vi "OnDrop.vi"(0 "XRef":T8, 1 "State In":T1 {"BlockNodeState"."Draw Style" items=["FunctionBlock", "ExpressVI", "Variable", "Elemental I/O", "32x32 Icon", "FunctionBlockCompact"]; "BlockNodeState"."Terminal Data"."Terminal Flags" format="%.0b"}) -> (14 "Reply":T6, 16 "State Out":T1 {"BlockNodeState"."Draw Style" items=["FunctionBlock", "ExpressVI", "Variable", "Elemental I/O", "32x32 Icon", "FunctionBlockCompact"]; "BlockNodeState"."Terminal Data"."Terminal Flags" format="%.0b"})   [LabVIEW 2018, in "N9010A_SCPI Node.xnode"]
uses:
  N9010A_SCPI Node.xnode
  <vilib>/XNodeSupport/XNodeXNodeRef.ctl
  State.ctl
  <vilib>/BlockNodeSupport/BlockNodeState.ctl
  <vilib>/BlockNodeSupport/TerminalData.ctl
  <vilib>/picture/picture.llb/imagedata.ctl
  Utility/command_spec.ctl
  <vilib>/XNodeSupport/XNodeStringArray.ctl
  <vilib>/XNodeSupport/XNodeString.ctl
  <vilib>/XNodeSupport/NI_XNodeSupport.lvlib
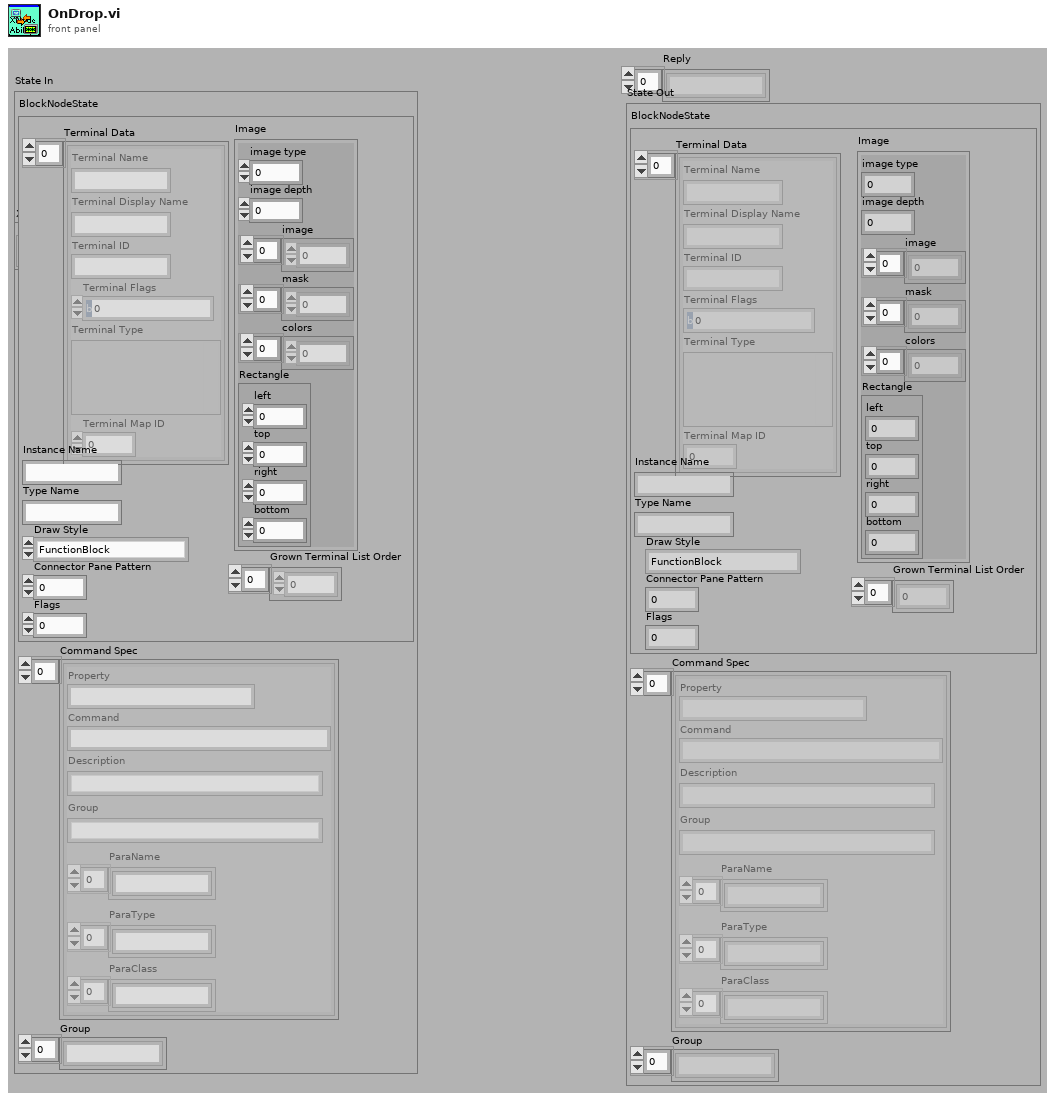
[diagram p1: front panel]
types:
  T1 = typedef "N9010A_SCPI Node.xnode/State.ctl" = cluster{"BlockNodeState":T2, "Command Spec":T5, "Group":string[]}
  T2 = typedef "BlockNodeState.ctl" = cluster{"Terminal Data":T3[], "Instance Name":string, "Type Name":string, "Draw Style":i32, "Connector Pane Pattern":i32, "Flags":i32, "Grown Terminal List Order":i32[], "Image":T4}
  T3 = typedef "TerminalData.ctl" = cluster{"Terminal Name":string, "Terminal Display Name":string, "Terminal ID":string, "Terminal Flags":i32, "Terminal Type":variant, "Terminal Map ID":i32}
  T4 = typedef "imagedata.ctl" = cluster{"image type":i32, "image depth":i32, "image":u8[], "mask":u8[], "colors":u32[], "Rectangle":cluster{"left":i16, "top":i16, "right":i16, "bottom":i16}}
  T5 = typedef "command_spec.ctl" = cluster{"Property":string, "Command":string, "Description":string, "Group":string, "ParaName":string[], "ParaType":string[], "ParaClass":string[]}[]
  T6 = typedef "NI_XNodeSupport.lvlib/XNodeStringArray.ctl" = T7[]
  T7 = typedef "NI_XNodeSupport.lvlib/XNodeString.ctl" = string
  T8 = typedef "NI_XNodeSupport.lvlib/XNodeXNodeRef.ctl" = refnum<vi>
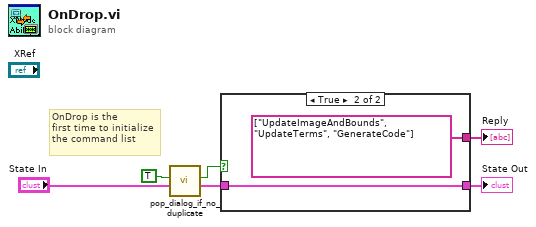
[diagram p0: block diagram]
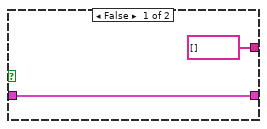
[diagram p2: hidden frame]
diagram:
  # "OnDrop is the\nfirst time to initialize\nthe command list"
  n1 = call "pop_dialog_if_no_duplicate.vi"("FirstTime"=TRUE, "State In in"="State In") -> ("NeedUpdate"=w1:bool, "State In out"=w4:T1)  [unwired: 7 in]
  n2 = case shown="True" w1 {
    tunnel: w4 -> [w8 w9]
    tunnel: [w8 w9] -> w5
    tunnel: [T6 [] ("Reply") T6 ["UpdateImageAndBounds", "UpdateTerms", "GenerateCode"] ("Reply")] -> w6
    frame False {
    }
    frame True {
    }
  }
  "Reply" <- w6
  "State Out" <- w5
